vi "PCO_SetFlimModulationParameter.vi"(8 "error in (no error)":errorcluster {"code" format="%x"}, 9 "wOutputWaveform":u16(ring) items=["none", "sine wave", "square wave"], 10 "wSourceSelect":u16(ring) items=["intern", "extern"], 11 "ph":u64) -> (0 "error out":errorcluster {"code" format="%x"}, 2 "ErrorMessage":i32 format="%x", 3 "ph out":u64)   [LabVIEW 2019, in "SDK.lvlib" / "SpecialCommandsFlim.lvlib"]
doc: "<b>Description:</b>\nThis function does set the modulation mode of the pco.flim. With this function the source of the modulation frequency signal can be selected and whether the signal is sent to the modulation output line <out – mod>. Furthermore the shape of the output waveform can be selected. No PCO_ArmCamera command is required to change these settings.\n\n<b>Supported camera type</b>\npco.flim\n\n<b>Descriptor dependency:</b>\nNone"
uses:
  SpecialCommandsFlim.lvlib
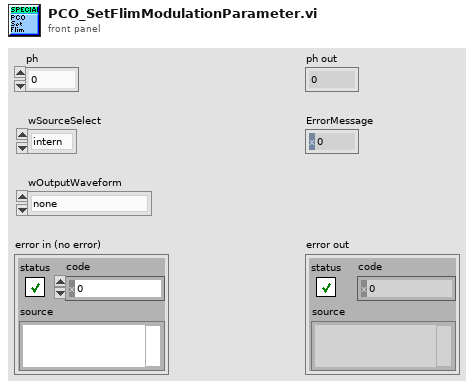
[diagram p1: front panel]
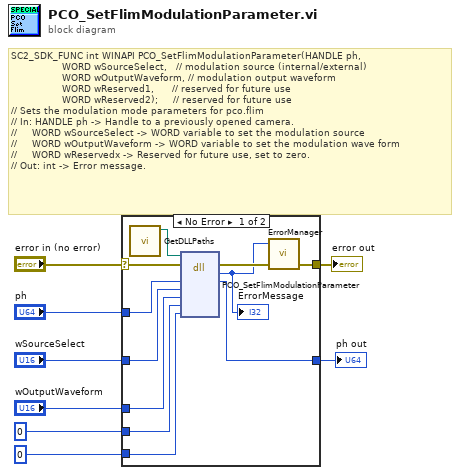
[diagram p0: block diagram]
diagram:
  # "SC2_SDK_FUNC int WINAPI PCO_SetFlimModulationParameter(HANDLE ph, \n                 WORD wSourceSelect,   // modulation source (internal/external)\n                 WORD wOutputWaveform, // modulation output waveform\n                 WORD wReserved1,      // reserved for future use\n                 WORD wReserved2);     // reserved for future use\n// Sets the modulation mode parameters for pco.flim\n// In: HANDLE ph -> Handle to a previously opened camera.\n//     WORD wSourceSelect -> WORD variable to set the modulation source\n//     WORD wOutputWaveform -> WORD variable to set the modulation wave form\n//     WORD wReservedx -> Reserved for future use, set to zero.\n// Out: int -> Error message."
  n1 = case shown="No Error" "error in (no error)" {
    selector: "error in (no error)" -> [w13 w21]
    tunnel: "ph" -> [w19 w20]
    tunnel: [w18 w20] -> w7
    tunnel: "wSourceSelect" -> [w17 _]
    tunnel: "wOutputWaveform" -> [w16 _]
    tunnel: [w12 w21] -> w4
    tunnel: u16 0 ("wReserved1") -> [w15 _]
    tunnel: u16 0 ("wReserved1") -> [w14 _]
    frame No Error {
      n2 = call "GetDLLPaths.vi"() -> ("SC2_Cam_Path"=w9:path)  [unwired: 9 in, 2 out]
      n3 = dll-call lib="?" fn="PCO_SetFlimModulationParameter"(path in=w9, error in=w13, "ph"=w19, "wSourceSelect"=w17, "wOutputWaveform"=w16, "wReserved1"=w15, "wReserved2"=w14) -> (error out=w11:errorcluster, "return type"=w10:i32, "ph"=w18:u64)  [unwired: 5 in, 1 out]
      "ErrorMessage" <- w10
      n4 = call "ErrorManager.vi"("error in (no error)"=w11, "error code"=w10) -> ("error out"=w12:errorcluster)  [unwired: 3 in]
    }
    frame Error {
    }
  }
  "ph out" <- w7
  "error out" <- w4
